vi "Get COM List.vi"(7 "To ASCII? (True)":bool=TRUE, 8 "error in (no error)":errorcluster) -> (0 "error out":errorcluster, 1 "raw string list":string, 2 "COM ports count":i32, 3 "COM list":T1[](array[typedef]))   [LabVIEW 2020, in "Get COM Descriptor.lvlib"]
doc: "Get list of available COM ports and their descriptors. Option To ASCII? will try to remove utf8 symbols (replaces accents with basic alphabet).\n\nDetails: https://github.com/smaslan/get-com-descriptor"
uses:
  Get COM Descriptor.lvlib
  COM port.ctl
  get_com_descriptor.dll
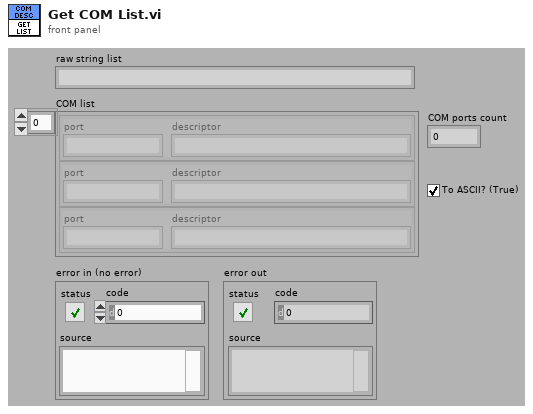
[diagram p1: front panel]
types:
  T1 = typedef "Get COM Descriptor.lvlib/COM port.ctl" = cluster{"port":string, "descriptor":string}
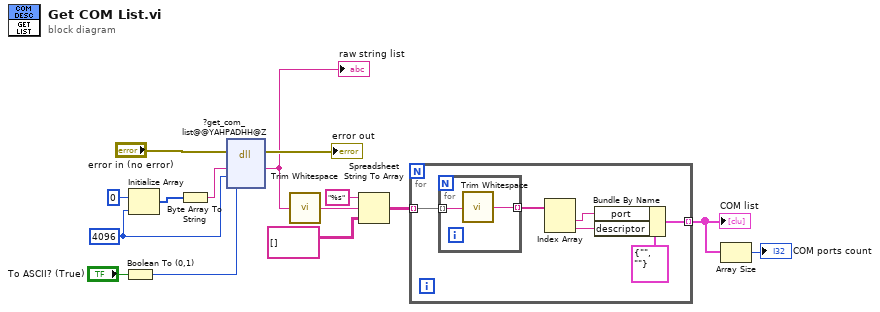
[diagram p0: block diagram]
diagram:
  w10 = 4096 ("dimension size")
  n1 = Boolean To (0,1)(Boolean="To ASCII? (True)") -> (0, 1=w1:i16)
  n2 = Initialize Array(u8 0 ("element"), w10) -> (w13:u8[])
  n3 = Byte Array To String(unsigned byte array=w13) -> (string=w11:string)
  n4 = dll-call lib="F:/Z_bridge_v4/other/get_com_descriptor/get_com_descriptor.dll" fn="?get_com_list@@YAHPADHH@Z"(error in="error in (no error)", "buf"=w11, "size"=w10, "to_ascii"=w1) -> (error out=→"error out":errorcluster, "buf"=w9:string)  [unwired: 5 in, 1 out]
  "raw string list" <- w9
  n5 = call <vilib>:"Trim Whitespace.vi"("string"=w9) -> ("trimmed string"=w8:string)  [unwired: 1 in]
  n6 = Spreadsheet String To Array(format string="%s", spreadsheet string=w8, array type (2D Dbl)=string[][] []) -> (array=w5:string[][])  [unwired: 1 in]
  n7 = for {
    tunnel: w5 -> [w21] mode=indexing
    tunnel: [w16] -> w4 mode=indexing
    n8 = for {
      tunnel: w21 -> [w23] mode=indexing
      tunnel: [w22] -> w20 mode=indexing
      n9 = call <vilib>:"Trim Whitespace.vi"("string"=w23) -> ("trimmed string"=w22:string)  [unwired: 1 in]
    }
    n10 = Index Array(array=w20) -> (element #1=w18:string, element #2=w17:string)  [unwired: 2 in]
    n11 = Bundle By Name(cluster=T1 {"port"="", "descriptor"=""} ("COM port"), "port"=w18, "descriptor"=w17) -> (w16:T1)
  }
  "COM list" <- w4
  n12 = Array Size(array=w4) -> (size(s)=→"COM ports count":i32)
